vi "test_Local Chassis Name Property.vi"(8 "error in (no error)":errorcluster, 11 "TestCase in":refnum<class "Scan Engine Scripting API Custom Device Unit Tests.lvclass">) -> (0 "error out":errorcluster, 3 "TestCase out":refnum<class "Scan Engine Scripting API Custom Device Unit Tests.lvclass">)   [LabVIEW 2019, in "Scan Engine Scripting API Custom Device Unit Tests.lvclass"]
uses:
  Scan Engine Scripting API Custom Device Unit Tests.lvclass
  <vilib>/addons/_JKI Toolkits/VI Tester/TestCase.llb/TestCase.lvclass
  Scripting/Scan Engine Scripting.lvlib
  Type Defs/Main Settings.ctl
  SEECD System Explorer.lvlib
  Type Defs/Local Chassis Settings.ctl
  C:/Program Files (x86)/National Instruments/LabVIEW 2019/vi.lib/addons/_JKI Toolkits/VI Tester/TestCase.llb/TestCase.lvclass
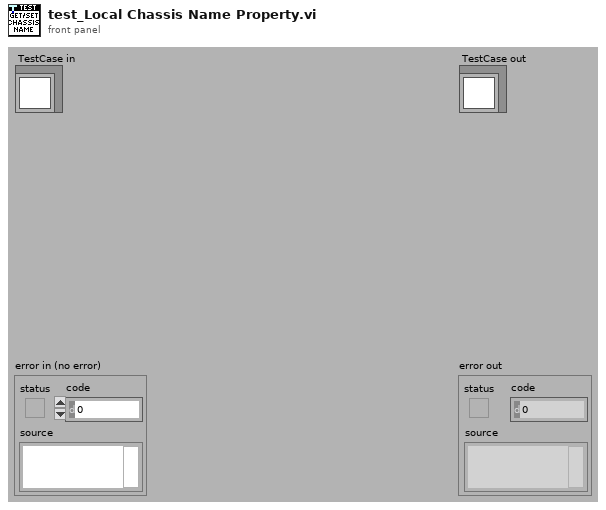
[diagram p1: front panel]
types:
  T1 = typedef "SEECD System Explorer.lvlib/Main Settings.ctl" = cluster{"sync to scan":bool, "scan engine decimation":u16, "delay after FPGA load (s)":u16}
  T2 = typedef "SEECD System Explorer.lvlib/Local Chassis Settings.ctl" = cluster{"name":string, "number of slots":i32}
  T3 = typedef "Custom Device API.lvlib/Custom Device Item Ref.ctl" = u64
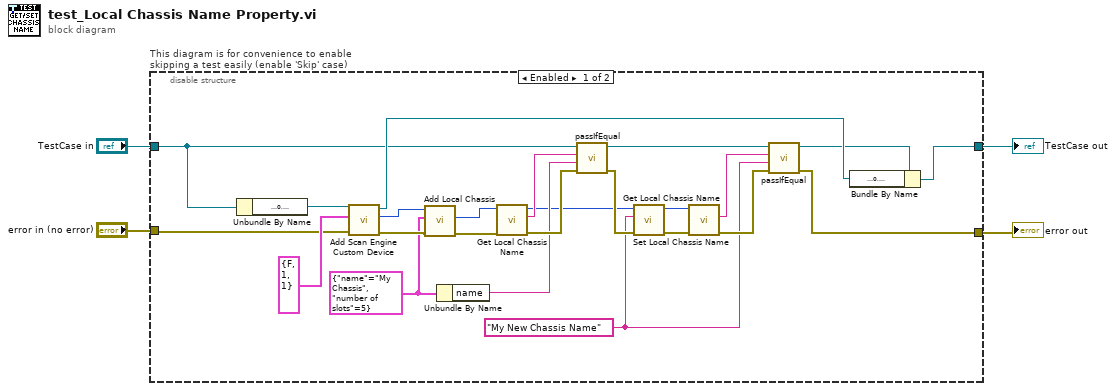
[diagram p0: block diagram]
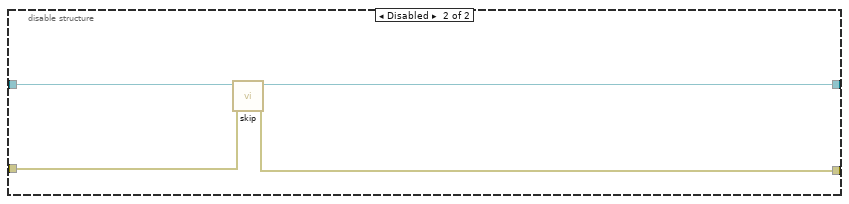
[diagram p2: hidden frame]
diagram:
  n1 = disable-structure "This diagram is for convenience to enable skipping a test easily (enable 'Skip' case)" shown="Enabled" {
    disable-tunnel: "TestCase in" -> [w18 w32]
    disable-tunnel: [w23 w30] -> w1
    disable-tunnel: [w5 w31] -> w3
    disable-tunnel: "error in (no error)" -> [w25 w29]
    frame Enabled {
      w8 = "My New Chassis Name" ("name")
      w22 = T2 {"name"="My Chassis", "number of slots"=5} ("settings")
      n2 = Unbundle By Name(w18) -> ("target ref"=w24:refnum<k24>)
      n3 = call "Add Scan Engine Custom Device.vi"("error in"=w25, "settings"=T1 {"sync to scan"=FALSE, "scan engine decimation"=1, "delay after FPGA load (s)"=1}, "target in"=w24) -> ("error out"=w27:errorcluster, "scan engine custom device ref"=w26:T3, "target out"=w19:refnum<k24>)  [unwired: 6 in]
      n4 = call "Add Local Chassis.vi"("error in"=w27, "settings"=w22, "scan engine custom device ref in"=w26) -> ("error out"=w20:errorcluster, "local chassis ref"=w21:T3)  [unwired: 4 in, 3 out]
      n5 = Unbundle By Name(w22) -> ("name"=w16:string)
      n6 = call "Get Local Chassis Name.vi"("error in"=w20, "chassis ref in"=w21) -> ("error out"=w17:errorcluster, "name"=w15:string, "chassis ref out"=w13:T3)  [unwired: 7 in]
      n7 = call-dynamic "passIfEqual.vi"("error in (no error)"=w17, "y"=w16, "x"=w15, "TestCase in"=w18) -> ("error out"=w14:errorcluster, "TestCase out"=w7:refnum<class "Scan Engine Scripting API Custom Device Unit Tests.lvclass">)  [unwired: 6 in]
      n8 = call "Set Local Chassis Name.vi"("error in"=w14, "name"=w8, "chassis ref in"=w13) -> ("error out"=w9:errorcluster, "chassis ref out"=w10:T3)  [unwired: 7 in]
      n9 = call "Get Local Chassis Name.vi"("error in"=w9, "chassis ref in"=w10) -> ("error out"=w11:errorcluster, "name"=w12:string)  [unwired: 7 in, 1 out]
      n10 = call-dynamic "passIfEqual.vi"("error in (no error)"=w11, "y"=w8, "x"=w12, "TestCase in"=w7) -> ("error out"=w5:errorcluster, "TestCase out"=w6:refnum<class "Scan Engine Scripting API Custom Device Unit Tests.lvclass">)  [unwired: 6 in]
      n11 = Bundle By Name(cluster=w6, "target ref"=w19) -> (w23:refnum<class "Scan Engine Scripting API Custom Device Unit Tests.lvclass">)
    }
    frame Disabled {
      # "skip test result while test is under development"
      n12 = call <vilib>:"skip.vi"("error in (no error)"=w29, "TestCase in"=w32) -> ("error out"=w31:errorcluster, "TestCase out"=w30:refnum<class "Scan Engine Scripting API Custom Device Unit Tests.lvclass">)  [unwired: 8 in]
    }
  }
  "error out" <- w3
  "TestCase out" <- w1
